vi "Verify FIFO Transfer Size with Host Buffer Depth.vi"(4 "Read/Write Size (samples)":u32, 6 "Host Buffer Depth (samples)":u32, 8 "error in":errorcluster) -> (0 "error out":errorcluster)   [LabVIEW 2016]
doc: "This VI verifies that the Host Buffer Depth is an integer multiple of the of the Read/Write Size."
uses:
  <vilib>/ErrorRing/Error Ring.xnode
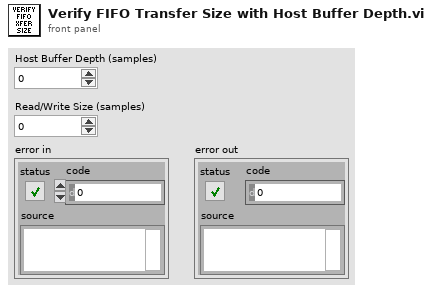
[diagram p1: front panel]
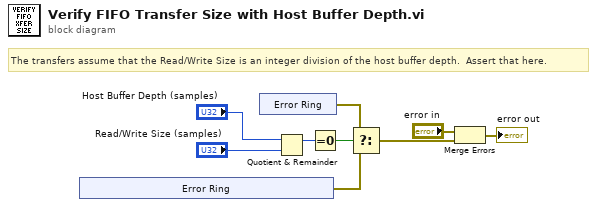
[diagram p0: block diagram]
diagram:
  # "The transfers assume that the Read/Write Size is an integer division of the host buffer depth.  Assert that here."
  n1 = xnode "Error Ring"() -> ("error out"=w6:errorcluster)
  n2 = xnode "Error Ring"() -> ("error out"=w5:errorcluster)
  n3 = Quotient & Remainder(x="Host Buffer Depth (samples)", y="Read/Write Size (samples)") -> (x-y*floor(x/y)=w8:u32)  [unwired: 1 out]
  n4 = Equal To 0?(x=w8) -> (x = 0?=w7:bool)
  n5 = Select(t=w5, s=w7, f=w6) -> (s? t:f=w1:errorcluster)
  n6 = Merge Errors("error in", w1) -> (→"error out":errorcluster)
